vi "BAM Generation Connections List_Actions.vi"(0 "Connection Cluster":T2 {"Packets"."Identifier" format="%08x"}, 1 "ref in":T4, 2 "State":T1=enum."Update", 7 "index":i32, 11 "error in (no error)":errorcluster) -> (3 "ref out":T4, 4 "Connections":T2[](array[typedef]) {"Packets"."Identifier" format="%08x"}, 8 "Connection Cluster Out":T2 {"Packets"."Identifier" format="%08x"}, 15 "error out":errorcluster {"code" min=0 max=0})   [LabVIEW 2013, in "J1939 Addon Engine.lvlib"]
uses:
  Engine/J1939 Addon Engine.lvlib
  Types/BAM Generation Connections List_Ref.ctl
  Types/BAM Generation Connection Cluster.ctl
  J1939 Utilities/Types/CAN Outgoing Message Cluster.ctl
  Types/TP Connections List State.ctl
  J1939 Utilities/J1939 Utilities.lvlib
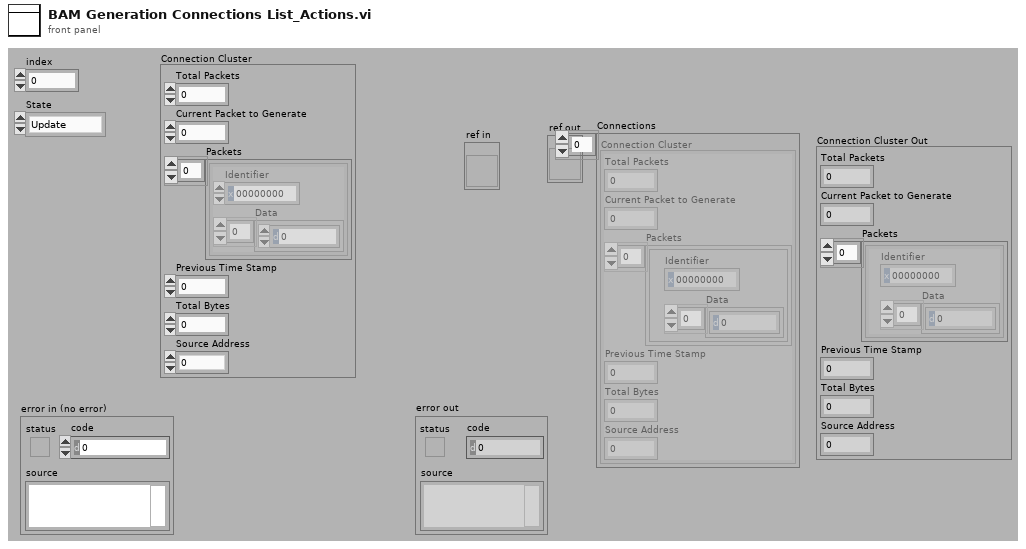
[diagram p1: front panel]
types:
  T1 = typedef "J1939 Addon Engine.lvlib/TP Connections List State.ctl" = enum16{"Add", "Update", "Get", "Remove", "Initialize"}
  T2 = typedef "J1939 Addon Engine.lvlib/BAM Generation Connection Cluster.ctl" = cluster{"Total Packets":u8, "Current Packet to Generate":u8, "Packets":T3[], "Previous Time Stamp":u32, "Total Bytes":u16, "Source Address":u8}
  T3 = typedef "J1939 Addon Shared.lvlib/J1939 Utilities.lvlib/CAN Outgoing Message Cluster.ctl" = cluster{"Identifier":u32, "Data":u8[]}
  T4 = typedef "J1939 Addon Engine.lvlib/BAM Generation Connections List_Ref.ctl" = refnum<vi>
  T5 = typedef "J1939 BAM Generation Connection Cluster.ctl" = cluster{"Total Packets":u8, "Current Packet to Generate":u8, "Packets":T6[], "Previous Time Stamp":u32, "Total Bytes":u16, "Source Address":u8}
  T6 = typedef "CAN Outgoing Message Cluster.ctl" = cluster{"Identifier":u32, "Data":u8[]}
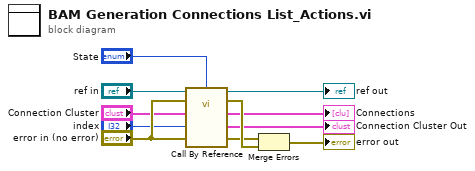
[diagram p0: block diagram]
diagram:
  n1 = call-by-ref "?"(reference="ref in", error in="error in (no error)", "Connection Cluster"="Connection Cluster", "State"="State", "index"="index", 11:"error in (no error)"="error in (no error)") -> (reference out=→"ref out":T4, error out=w10:errorcluster, "Connections"=→"Connections":T5[], "Connection Cluster Out"=→"Connection Cluster Out":T5, 15:"error out"=w9:errorcluster)  [unwired: 9 in]
  n2 = Merge Errors(w9, w10) -> (→"error out":errorcluster)
